vi "Rolling Average Floder.vi"() -> ()   [LabVIEW 2015]
doc: "The Low-Level Ring Rolling Average VI shows how to compute a rolling average while performing a ring acquisition. A queue is used to keep track of the image references used in the average. Once the queue becomes full, the oldest image reference is removed and released from the ring buffer.\n\nThis example requires NI Vision Development Module."
uses:
  <vilib>/vision/Image Controls.llb/IMAQ Image.ctl
  <vilib>/Utility/error.llb/DialogType.ctl
  <vilib>/vision/NI_Vision_Development_Module.lvlib
panel:
  out "数值":i32
  out "Display":T1(plugin-control)
  in  "Images Folder":path=path "F:/Data/160306 HeartBeating"
  in  "Number of Images to Average":i32=5
  out "Rolling Average":T1(plugin-control)
  in  "Stop":bool
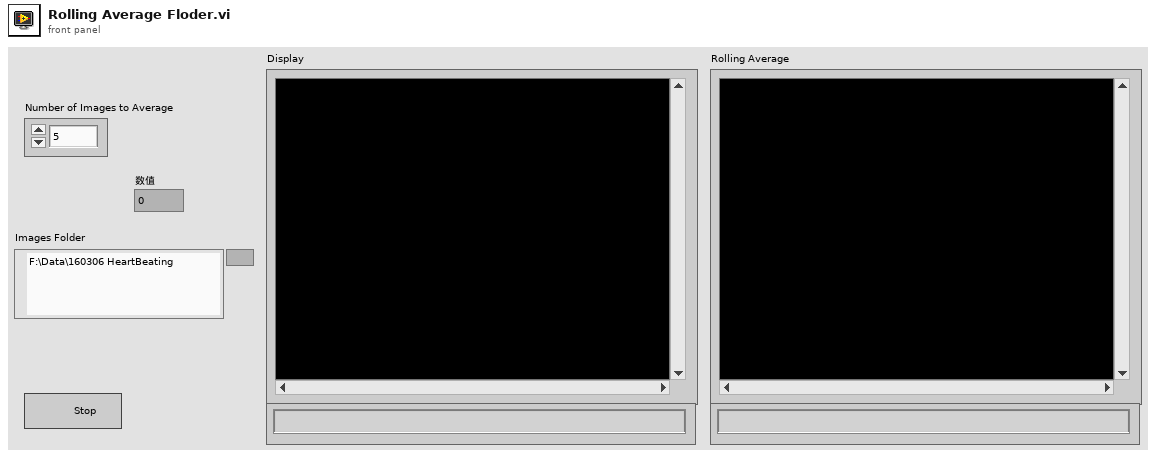
[diagram p1: front panel]
types:
  T1 = typedef "IMAQ Image.ctl" = refnum<image>
  T2 = typedef "Image Type" = u32
  T3 = typedef "DialogType.ctl" = u16
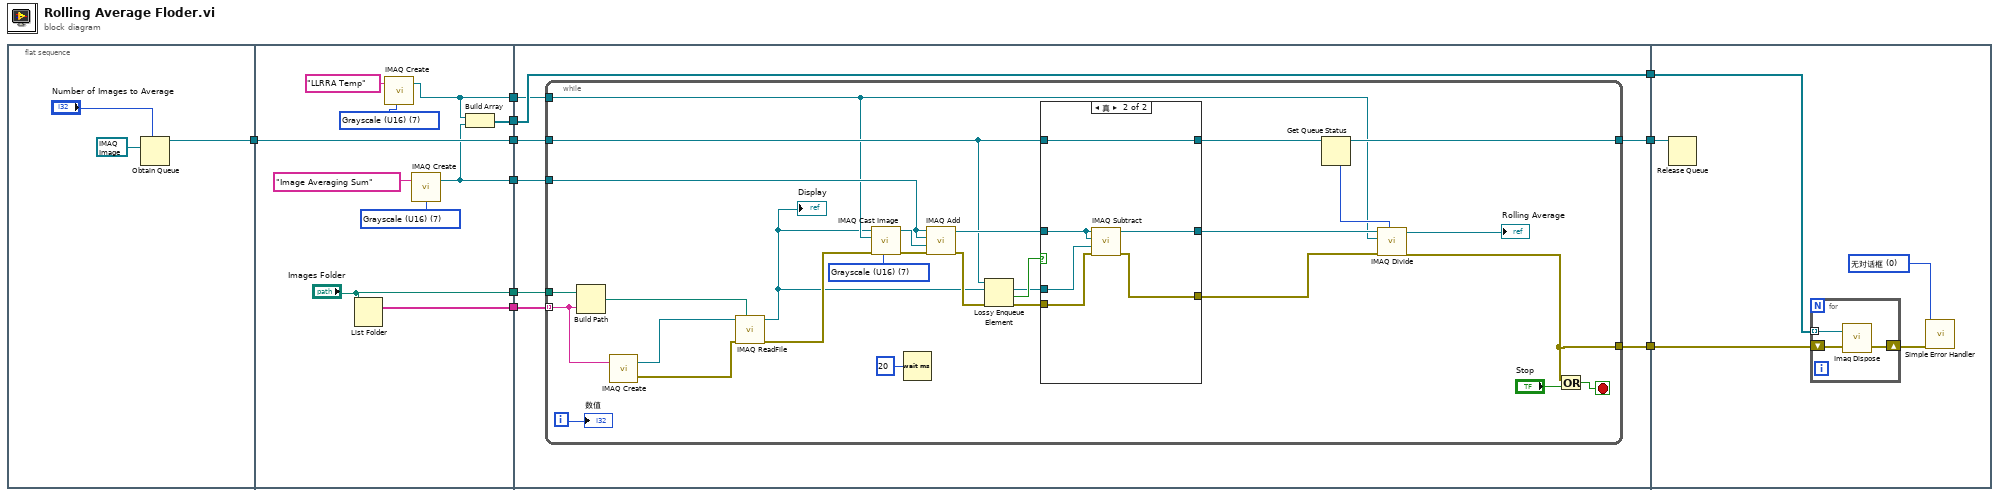
[diagram p0: block diagram]
diagram:
  n1 = flat-sequence {
    tunnel: [w12] -> w10
    tunnel: w10 -> [w23]
    tunnel: [w23] -> w9
    tunnel: [w17] -> w8
    tunnel: [w18] -> w5
    tunnel: [w16] -> w3
    tunnel: [w15] -> w2
    tunnel: ["Images Folder"] -> w1
    tunnel: w9 -> [w30]
    tunnel: w8 -> [w29]
    tunnel: [w24] -> w7
    tunnel: [w28] -> w6
    tunnel: w5 -> [w31]
    tunnel: [w31] -> w4
    tunnel: w3 -> [w27]
    tunnel: w2 -> [w25]
    tunnel: w1 -> [w26]
    tunnel: w7 -> [w71]
    tunnel: w6 -> [w74]
    tunnel: w4 -> [w72]
    frame #0 {
      n2 = Obtain Queue(max queue size (-1, unlimited)="Number of Images to Average", element data type=T1 refnum ("New Image")) -> (queue out=w12:refnum<queue>)  [unwired: 3 in, 2 out]
    }
    frame #1 {
      w20 = T2 7 items=["Grayscale (U8)", "Grayscale (I16)", "Grayscale (SGL)", "Complex (CSG)", "RGB (U32)", "HSL (U32)", "RGB (U64)", "Grayscale (U16)"] ("Image Type")
      w21 = T2 7 items=["Grayscale (U8)", "Grayscale (I16)", "Grayscale (SGL)", "Complex (CSG)", "RGB (U32)", "HSL (U32)", "RGB (U64)", "Grayscale (U16)"] ("Image Type")
      n3 = List Folder(path="Images Folder") -> (filenames=w15:string[])  [unwired: 1 in, 5 out]
      n4 = call "IMAQ Create"("Image Name"="LLRRA Temp", "Image Type"=w20) -> ("New Image"=w16:T1)  [unwired: 3 in, 1 out]
      n5 = call "IMAQ Create"("Image Name"="Image Averaging Sum", "Image Type"=w21) -> ("New Image"=w17:T1)  [unwired: 3 in, 1 out]
      n6 = Build Array(w16, w17) -> (w18:T1[])
    }
    frame #2 {
      n7 = while {
        tunnel: w30 -> [w55]
        tunnel: w29 -> [w49]
        tunnel: [w50] -> w28
        tunnel: w27 -> [w45]
        tunnel: w26 -> [w44]
        tunnel: w25 -> [w36] mode=indexing
        tunnel: [w32] -> w24
        i -> [w40]
        stop <- w51 stop-if-true
        w47 = T2 7 items=["Grayscale (U8)", "Grayscale (I16)", "Grayscale (SGL)", "Complex (CSG)", "RGB (U32)", "HSL (U32)", "RGB (U64)", "Grayscale (U16)"] ("Image Type")
        n8 = Build Path(base path=w44, name or relative path=w36) -> (appended path=w43:path)
        n9 = call "IMAQ Create"("Image Name"=w36) -> ("New Image"=w35:T1, "error out"=w34:errorcluster)  [unwired: 3 in, 1 out]
        n10 = call "IMAQ ReadFile"("File Path"=w43, "error in (no error)"=w34, "Image"=w35) -> ("error out"=w42:errorcluster, "Image Out"=w37:T1)  [unwired: 2 in, 5 out]
        "Display" <- w37
        n11 = call "IMAQ Cast Image"("Image Type"=w47, "error in (no error)"=w42, "Image Dst"=w45, "Image Src"=w37) -> ("error out"=w48:errorcluster, "Image Dst Out"=w38:T1)  [unwired: 6 in]
        n12 = Wait (ms)(milliseconds to wait=u32 20 ("等待时间（毫秒）")) -> ()  [unwired: 1 out]
        n13 = call "IMAQ Add"("Image Src A"=w49, "Image Dst"=w49, "Image Src B"=w38, "error in (no error)"=w48) -> ("Image Dst Out"=w57:T1, "error out"=w60:errorcluster)  [unwired: 3 in]
        n14 = Lossy Enqueue Element(queue=w55, element=w37, error in (no error)=w60) -> (overflow element=w58:T1, overflow?=w59:bool, error out=w56:errorcluster)  [unwired: 1 out]
        n15 = case shown="真" w59 {
          tunnel: w58 -> [_ w68]
          tunnel: w57 -> [w62 w65]
          tunnel: w56 -> [w63 w69]
          tunnel: [w63 w66] -> w39
          tunnel: [w62 w64] -> w46
          tunnel: [w61 w67] -> w54
          tunnel: w55 -> [w61 w67]
          frame False {
          }
          frame True {
            n16 = call "IMAQ Subtract"("Image Src A"=w65, "Image Dst"=w65, "Image Src B"=w68, "error in (no error)"=w69) -> ("Image Dst Out"=w64:T1, "error out"=w66:errorcluster)  [unwired: 3 in]
          }
        }
        n17 = Get Queue Status(queue=w54) -> (queue out=w50:refnum<queue>, # elements in queue=w53:i32)  [unwired: 2 in, 6 out]
        n18 = call "IMAQ Divide"("Image Src A"=w46, "Constant"=w53, "Image Dst"=w45, "error in (no error)"=w39) -> ("Image Dst Out"=→"Rolling Average":T1, "error out"=w32:errorcluster)  [unwired: 3 in]
        n19 = Or(x=w32, y="Stop") -> (x .or. y?=w51:bool)
        "数值" <- w40
      }
    }
    frame #3 {
      w70 = T3 0 items=["无对话框", "确定信息", "继续或停止信息", "确定信息＋警告", "继续/停止+警告"] ("type of dialog (OK msg:1)")
      n20 = Release Queue(queue=w74) -> ()  [unwired: 2 in, 3 out]
      n21 = for {
        shift-right: [w76] -> w73
        shift-left: w71 -> [w77]
        tunnel: w72 -> [w75] mode=indexing
        n22 = call "Imaq Dispose"("Image"=w75, "error in (no error)"=w77) -> ("error out"=w76:errorcluster)  [unwired: 4 in]
      }
      n23 = call <vilib>:"Simple Error Handler.vi"("type of dialog (OK msg:1)"=w70, "error in (no error)"=w73) -> ()  [unwired: 3 in, 5 out]
    }
  }
